vi "setUp.vi"(8 "error in":errorcluster, 11 "reference in":refnum<class "Deployment.lvclass">) -> (0 "error out":errorcluster, 3 "reference out":refnum<class "Deployment.lvclass">)   [LabVIEW 2020, in "Deployment.lvclass"]
doc: "setUp runs prior to the test method during test execution. Use this method to initialize any object data required by your tests."
uses:
  Deployment.lvclass
  C:/Program Files (x86)/National Instruments/LabVIEW 2020/vi.lib/addons/_JKI Toolkits/VI Tester/TestCase.llb/TestCase.lvclass
  Deployment.lvclass/Deployment.ctl
  <vilib>/addons/_JKI Toolkits/VI Tester/TestCase.llb/TestCase.lvclass
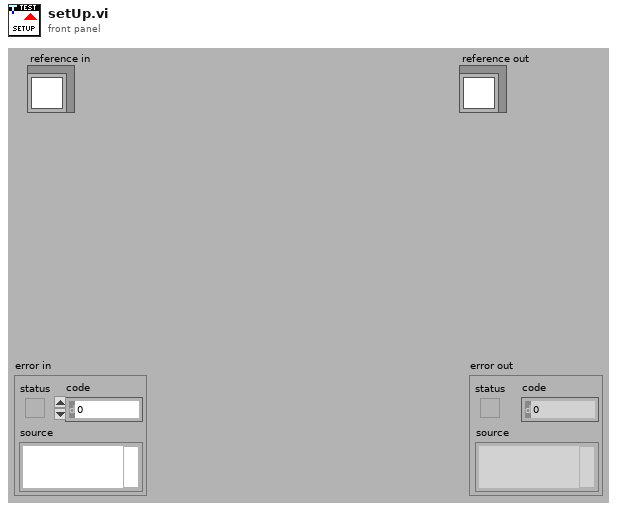
[diagram p1: front panel]
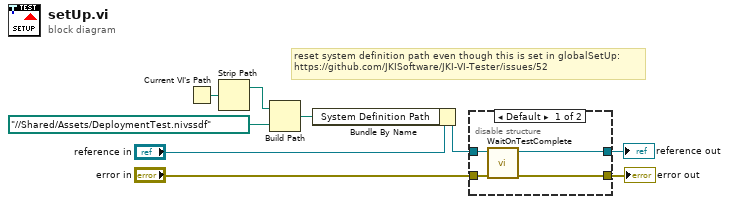
[diagram p0: block diagram]
diagram:
  # "reset system definition path even though this is set in globalSetUp:\nhttps://github.com/JKISoftware/JKI-VI-Tester/issues/52"
  n1 = Current VI's Path() -> (path=w6:path)
  n2 = Strip Path(path=w6) -> (stripped path=w3:path)  [unwired: 1 out]
  n3 = Build Path(base path=w3, name or relative path=path "../../Shared/Assets/DeploymentTest.nivssdf" ("System Definition Name")) -> (appended path=w1:path)
  n4 = Bundle By Name(cluster="reference in", "System Definition Path"=w1) -> (w4:refnum<class "Deployment.lvclass">)
  n5 = disable-structure shown="Default" {
    disable-tunnel: "error in" -> [w13 w14]
    disable-tunnel: [w12 w14] -> w9
    disable-tunnel: [w11 w15] -> w8
    disable-tunnel: w4 -> [w10 w15]
    frame condition #0 (active) {
      n6 = call <vilib>:"WaitOnTestComplete.vi"("error in (no error)"=w13, "TestCase in"=w10) -> ("error out"=w12:errorcluster, "TestCase out"=w11:refnum<class "Deployment.lvclass">)  [unwired: 8 in]
    }
    frame condition #1 {
    }
  }
  "error out" <- w9
  "reference out" <- w8
